vi "Close.vi"(8 "error in (no error)":errorcluster, 11 "DeviceRefnum":u64) -> (0 "error out":errorcluster, 2 "function return":i32)   [LabVIEW 2016]
doc: "Closes the RTLSDR resource.\nIf this is not called upon terminating the application, the resource remains in memory. It will not be possible to open the resource again unless the rtlsdr is undplugged and replugged, or the system is restarted."
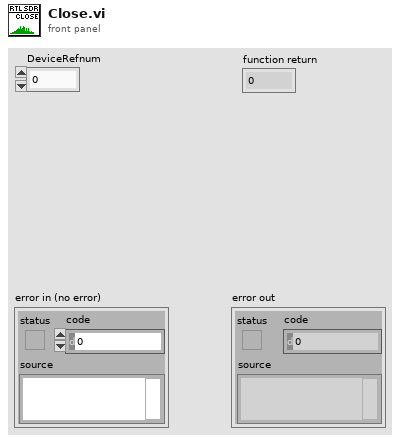
[diagram p1: front panel]
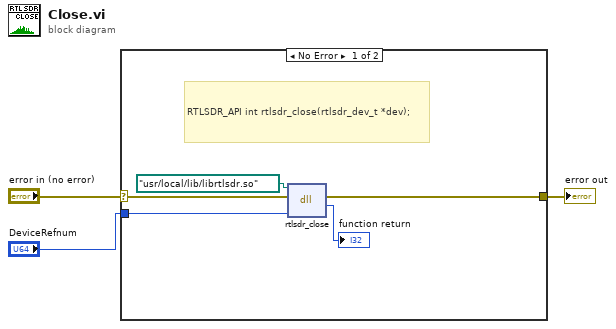
[diagram p0: block diagram]
diagram:
  n1 = case shown="No Error" "error in (no error)" {
    selector: "error in (no error)" -> [w6 w9]
    tunnel: [w5 w9] -> w3
    tunnel: "DeviceRefnum" -> [w8 _]
    frame No Error {
      # "RTLSDR_API int rtlsdr_close(rtlsdr_dev_t *dev);"
      n2 = dll-call lib="C:/Program Files (x86)/National Instruments/LabVIEW 2016/vi.lib/rtlsdr/rtlsdr.*" fn="rtlsdr_close"(path in=path "/usr/local/lib/librtlsdr.so", error in=w6, "DeviceRefnum"=w8) -> (error out=w5:errorcluster, "return type"=→"function return":i32)  [unwired: 2 in, 1 out]
    }
    frame Error {
    }
  }
  "error out" <- w3
